vi "AbortGeneration.vi"(8 "error in (no error)":errorcluster, 11 "IviFgen in":refnum<class "IviFgen.lvclass">) -> (0 "error out":errorcluster, 3 "IviFgen out":refnum<class "IviFgen.lvclass">)   [LabVIEW 2014, in "FgenPlugins.lvlib" / "IviFgen.lvclass"]
uses:
  IviFgen.lvclass
  FgenPluginBaseClass/FgenPluginsBase.lvclass/FgenPluginsBase.ctl
  FgenPluginBaseClass/Accessors/Read Channels.vi
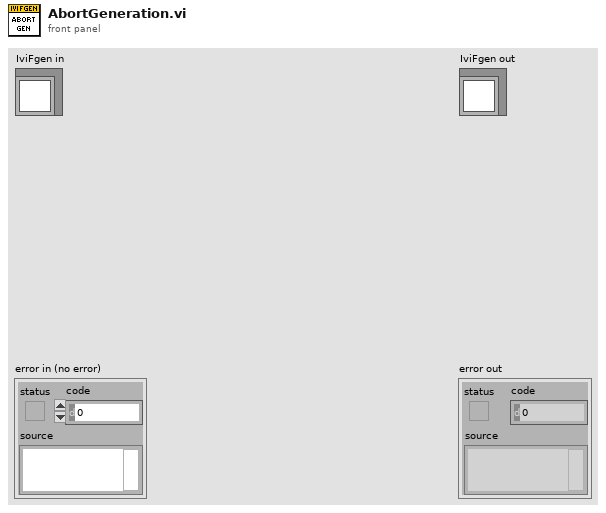
[diagram p1: front panel]
types:
  T1 = typedef "Channel.ctl" = cluster{"Name":string, "Enabled":bool, "Operation":enum16{"Continuous", "Burst"}, "Impedance (50)":dbl, "Handle":string, "Connected":bool, "Mode (Function)":enum16{"Function", "Arbitrary", "Sequence"}}
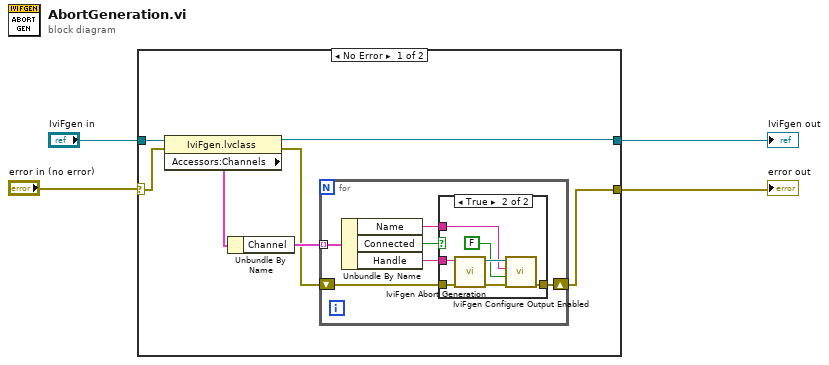
[diagram p0: block diagram]
diagram:
  n1 = case shown="No Error" "error in (no error)" {
    selector: "error in (no error)" -> [w10 w27]
    tunnel: [w6 w27] -> w3
    tunnel: [w5 w26] -> w1
    tunnel: "IviFgen in" -> [w11 w26]
    frame No Error {
      n2 = property class="IviFgen.lvclass"(reference=w11, error in=w10) -> (reference out=w5:refnum<class "IviFgen.lvclass">, error out=w7:errorcluster, "Accessors:Channels"=w9:cluster{"Count":u16, "Channel":T1[]})
      n3 = Unbundle By Name(w9) -> ("Channel"=w8:T1[])
      n4 = for {
        tunnel: w8 -> [w17] mode=indexing
        shift-right: [w13] -> w6
        shift-left: w7 -> [w14]
        n5 = Unbundle By Name(w17) -> ("Name"=w12:string, "Connected"=w16:bool, "Handle"=w15:string)
        n6 = case shown="True" w16 {
          tunnel: w15 -> [_ w25]
          tunnel: w14 -> [w18 w24]
          tunnel: [w18 w21] -> w13
          tunnel: w12 -> [_ w20]
          frame False {
          }
          frame True {
            n7 = call <vilib>:"IviFgen Abort Generation.vi"("error in (no error)"=w24, "instrument handle"=w25) -> ("error out"=w23:errorcluster, "instrument handle out"=w22:refnum<k15>)  [unwired: 8 in]
            n8 = call <vilib>:"IviFgen Configure Output Enabled.vi"("error in (no error)"=w23, "channel enabled (True)"=FALSE, "channel name (\"CHANNEL1\")"=w20, "instrument handle"=w22) -> ("error out"=w21:errorcluster)  [unwired: 6 in, 1 out]
          }
        }
      }
    }
    frame Error {
    }
  }
  "error out" <- w3
  "IviFgen out" <- w1
